vi "TestTactic.vi"(8 "error in (no error)":errorcluster, 9 "Game in":refnum<class "Game.lvclass">, 10 "Robot":refnum<class "Robot.lvclass">, 11 "Tactic in":refnum<class "TestTactic.lvclass">) -> (0 "error out":errorcluster, 2 "Robot out":refnum<class "Robot.lvclass">, 3 "Tactic out":refnum<class "TestTactic.lvclass">)   [LabVIEW 2023, in "TestTactic.lvclass"]
uses:
  TestTactic.lvclass
  Robot_class/Robot.lvclass
  Game_class/Game.lvclass
  States.ctl
  Robot_class/tactics.ctl
  Tactic_class/Tactic.lvclass/Tactic.ctl
  TestTactic.lvclass/TestTactic.ctl
  Robot_class/Robot.lvclass/Robot.ctl
  Tactic_class/Read Skillbook.vi
  Robot_class/Write tactic.vi
  Write States.vi
  Skillbook_class/Skillbook.lvclass
  DefBallEnemySkill_class/DefBallEnemySkill.lvclass
panel:
  out "x .or. y?":bool
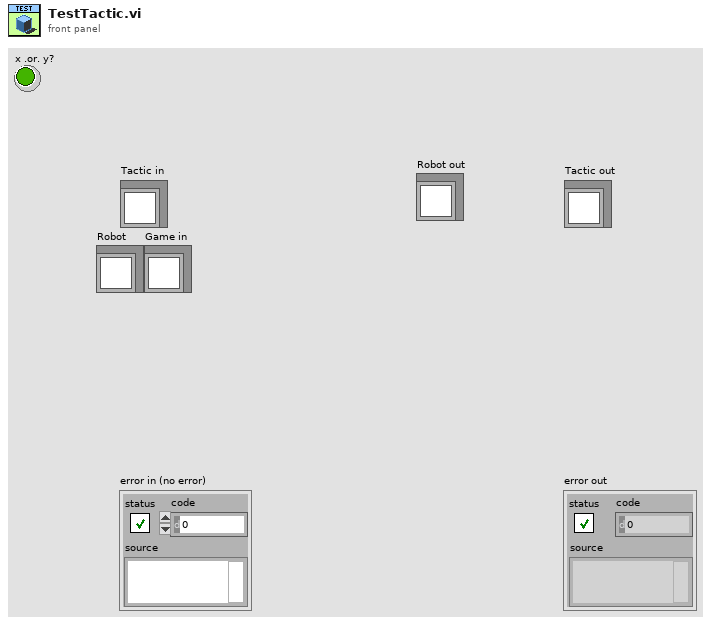
[diagram p1: front panel]
types:
  T1 = typedef "tactics.ctl" = enum16{"ReceivePassInFuturePoint", "Roller", "PrepareRollToPassRollerGoTo", "PrepareRollToPassReceiverGoTo", "WaitRoll", "PositionToRoll", "PenaltyAttacker", "PassObserver", "PenaltyDefense", "TableReceiverTactic", "Test", "DefendGoal", "Marker", "FollowAttacker", "DefendArea", "Shoot", "AttackerAimGoal", "AttackerBallOutOfField", "AttackerBlock", "AttackerStop", "Duelist", "Halt", "ZigZag", "GoTo", "Timeout", "KickToPassReceiver", "PositionToReceivePass", "DefendAreaVSS", "DefendGoalVSS", "KickVSS", "AttackVSS", "DispBallVSS", "PenaltyAttackVSS", "WaitPass"}
  T2 = typedef "States.ctl" = enum16{"State 1", "Exit"}
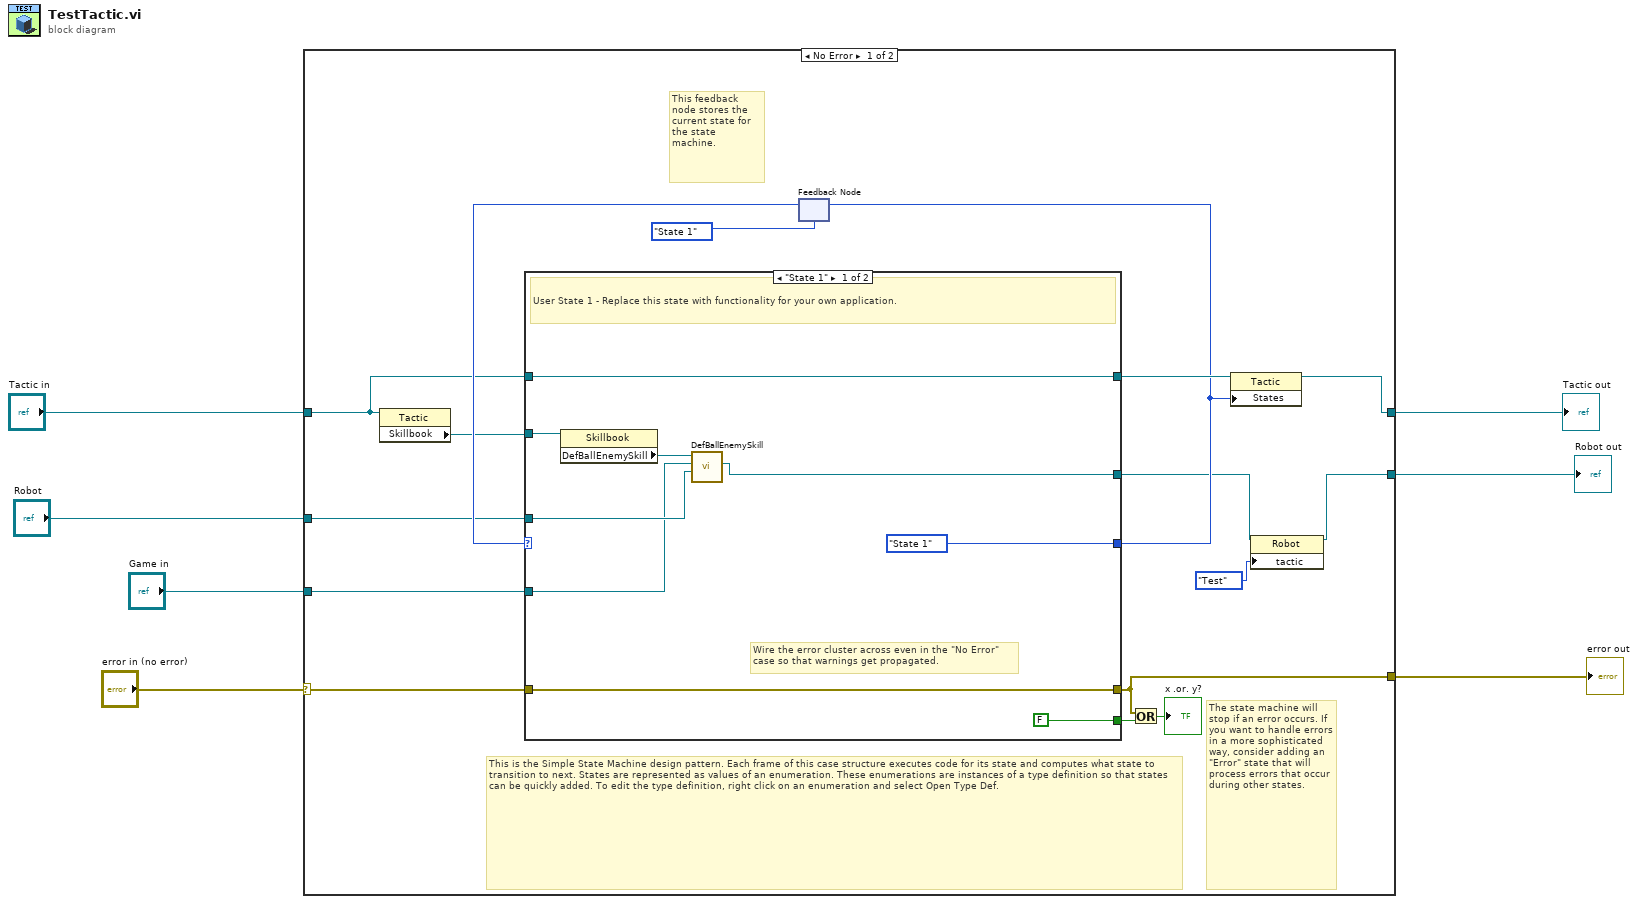
[diagram p0: block diagram]
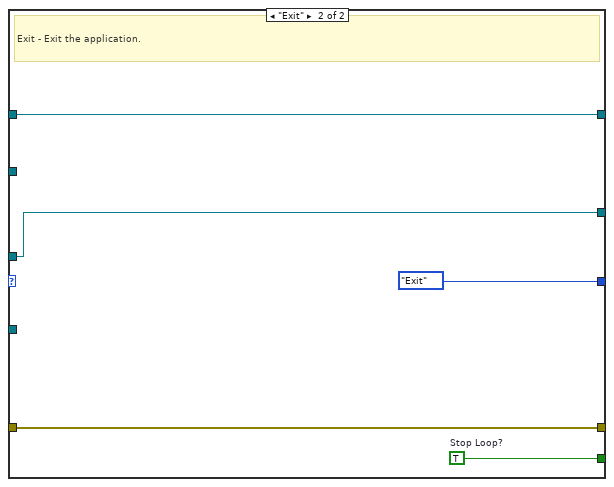
[diagram p2: hidden frame]
diagram:
  n1 = case shown="No Error" "error in (no error)" {
    selector: "error in (no error)" -> [w20 w40]
    tunnel: [w19 w40] -> w6
    tunnel: [w13 w39] -> w5
    tunnel: "Tactic in" -> [w16 w39]
    tunnel: "Robot" -> [w17 w38]
    tunnel: [w8 w38] -> w3
    tunnel: "Game in" -> [w11 _]
    frame No Error {
      # "The state machine will stop if an error occurs. If you want to handle errors in a more sophisticated way, consider adding an \"Error\" state that will process errors that occur during other states."
      # "This feedback node stores the current state for the state machine."
      # "This is the Simple State Machine design pattern. Each frame of this case structure executes code for its state and computes what state to transition to next. States are represented as values of an enumeration. These enumerations are instances of a type definition so that states can be quickly added. To edit the type definition, right click on an enumeration and select Open Type Def."
      # "Wire the error cluster across even in the \"No Error\"\ncase so that warnings get propagated."
      n2 = property class="Tactic"(reference=w16) -> ("Skillbook"=w15:refnum<class "Skillbook.lvclass">)  [unwired: 1 in, 2 out]
      n3 = feedback #1(States."State 1" ("States")) -> (w21:T2)
      n4 = case shown="\"State 1\"" w21 {
        tunnel: [States."State 1" ("States") States."Exit" ("States")] -> w12
        tunnel: [FALSE ("Stop Loop?") w37] -> w23
        tunnel: w20 -> [w31 w36]
        tunnel: [w31 w36] -> w19
        tunnel: w15 -> [w29 _]
        tunnel: w17 -> [w26 w34]
        tunnel: [w25 w34] -> w9
        tunnel: [w28 w33] -> w14
        tunnel: w16 -> [w28 w33]
        tunnel: w11 -> [w24 _]
        frame "State 1" {
          # "User State 1 - Replace this state with functionality for your own application."
          n5 = property class="Skillbook"(reference=w29) -> ("DefBallEnemySkill"=w27:refnum<class "DefBallEnemySkill.lvclass">)  [unwired: 1 in, 2 out]
          n6 = call "DefBallEnemySkill.vi"("Robot"=w26, "Game"=w24, "DefBallEnemySkill in"=w27) -> ("robot out"=w25:refnum<class "Robot.lvclass">)  [unwired: 6 in, 2 out]
        }
        frame "Exit" {
          w37 = TRUE  # Stop Loop?
          # "Exit - Exit the application."
        }
      }
      n7 = feedback-in #1(w12) -> ()
      n8 = Or(x=w19, y=w23) -> (x .or. y?=→"x .or. y?":bool)
      n9 = property class="Tactic"(reference=w14, "States"=w12) -> (reference out=w13:refnum<class "TestTactic.lvclass">)  [unwired: 1 in, 1 out]
      n10 = property class="Robot"(reference=w9, "tactic"=tactics."Test") -> (reference out=w8:refnum<class "Robot.lvclass">)  [unwired: 1 in, 1 out]
    }
    frame Error {
    }
  }
  "error out" <- w6
  "Tactic out" <- w5
  "Robot out" <- w3
